vi "Slack-Dialog.vi"(0 "Cluster In":cluster{"Numeric":dbl}, 7 "AppName":string="Slack Demo") -> (4 "Cluster out":cluster{"Numeric":dbl}, 8 "Canceled?":bool)   [LabVIEW 2015]
uses:
  Controls/KBackground Gradient/KBackground Gradient.xctl
panel:
  in  "Gradient":dbl(xcontrol)
  in  "Tab":enum32{"Page 1", "Page 2"}(tab)
  out "Channel":string
  out "Workspace":string
  out "Users":i32(listbox) caption="channel"
  in  "Refresh Button":bool
  in  "Sign in Button":bool
  in  "Cancel":bool
  in  "OK":bool
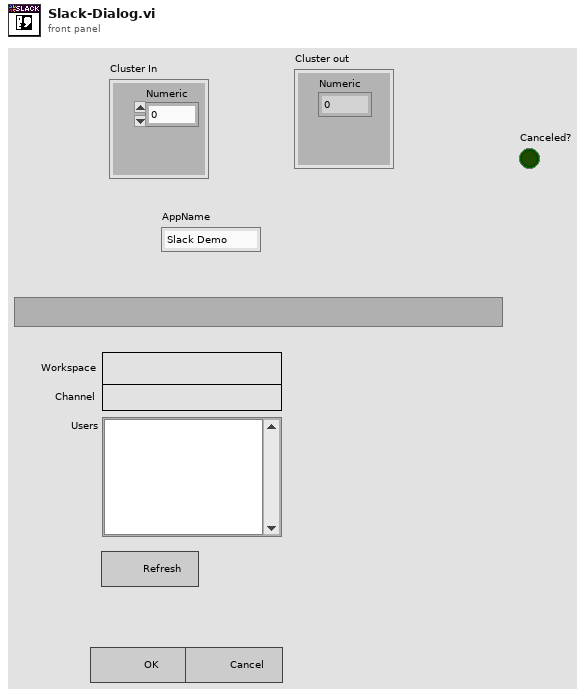
[diagram p1: front panel]
types:
  T1 = typedef "Slack-Configuration.ctl" = cluster{"app_id":string, "authed_user":cluster{"id":string}, "access_token":string, "bot_user_id":string, "team":cluster{"id":string, "name":string}, "bot channel":cluster{"id":string, "name":string}}
  T2 = typedef "Slack-User.ctl" = cluster{"id":string, "name":string}
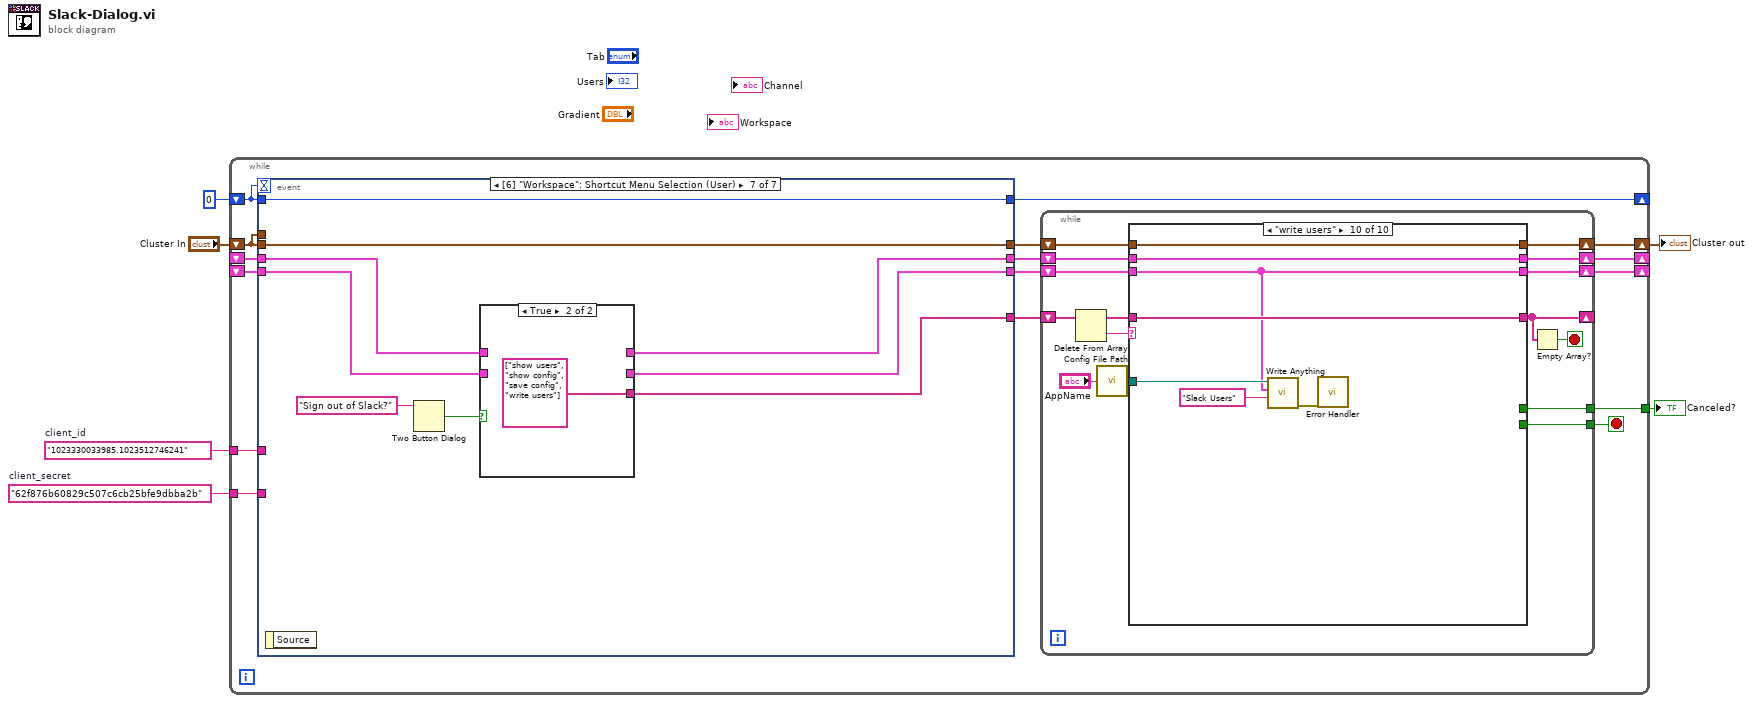
[diagram p0: block diagram]
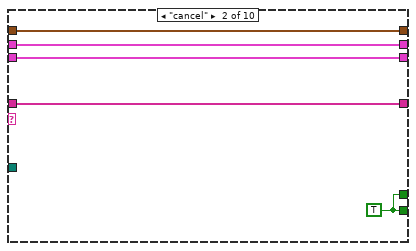
[diagram p3: hidden frame]
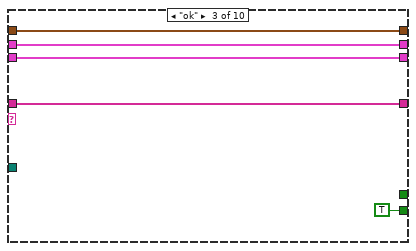
[diagram p4: hidden frame]
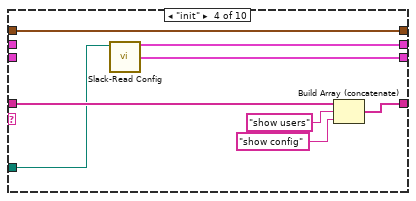
[diagram p5: hidden frame]
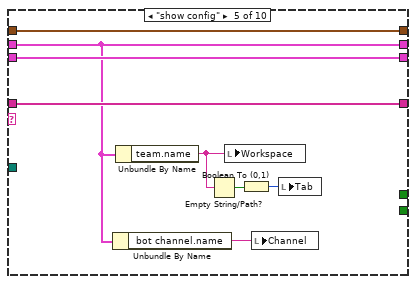
[diagram p6: hidden frame]
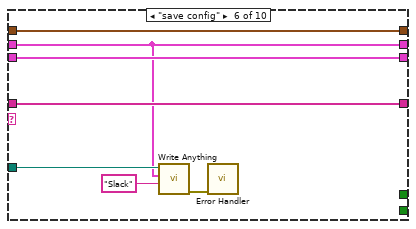
[diagram p7: hidden frame]
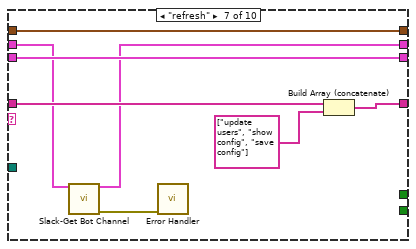
[diagram p8: hidden frame]
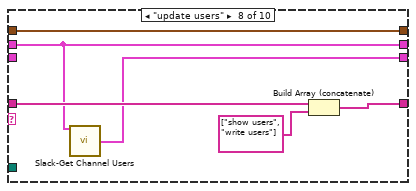
[diagram p9: hidden frame]
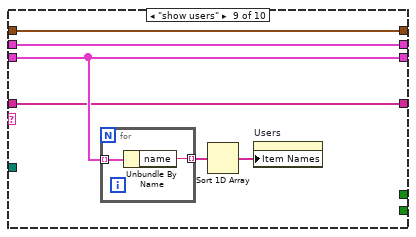
[diagram p10: hidden frame]
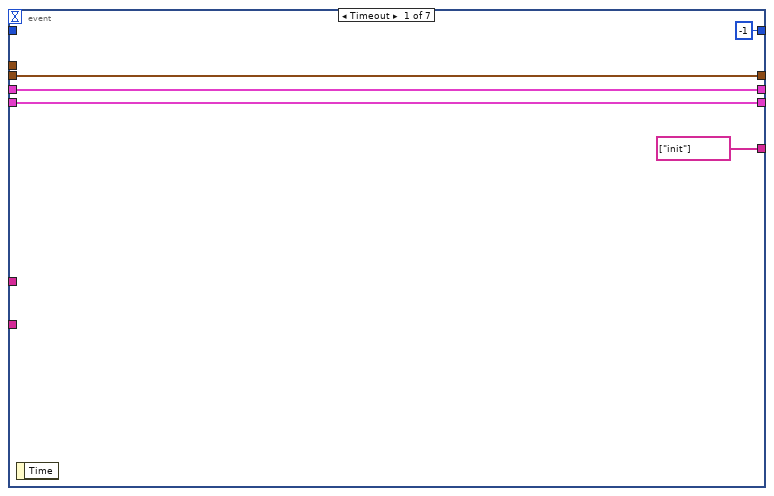
[diagram p11: hidden frame]
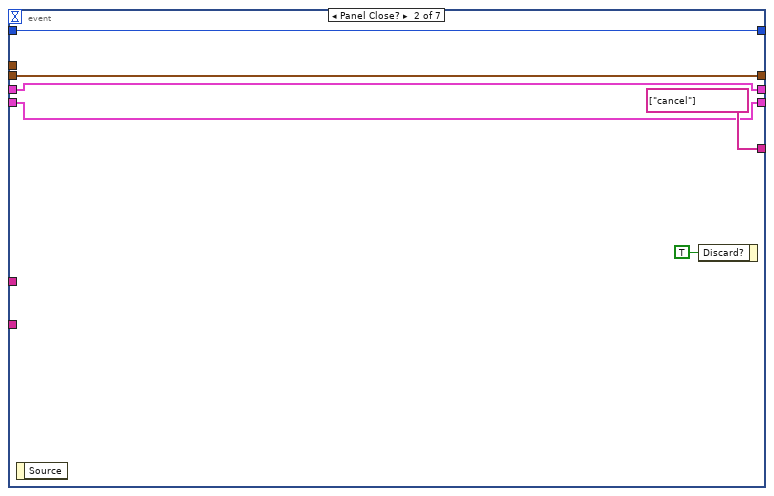
[diagram p12: hidden frame]
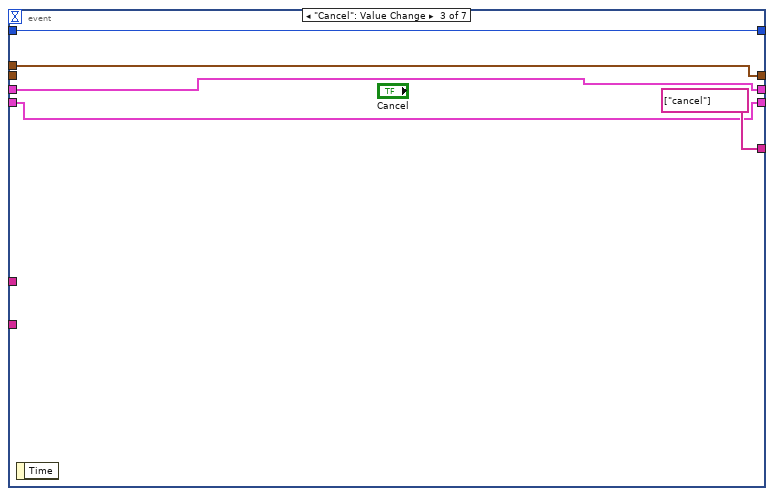
[diagram p13: hidden frame]
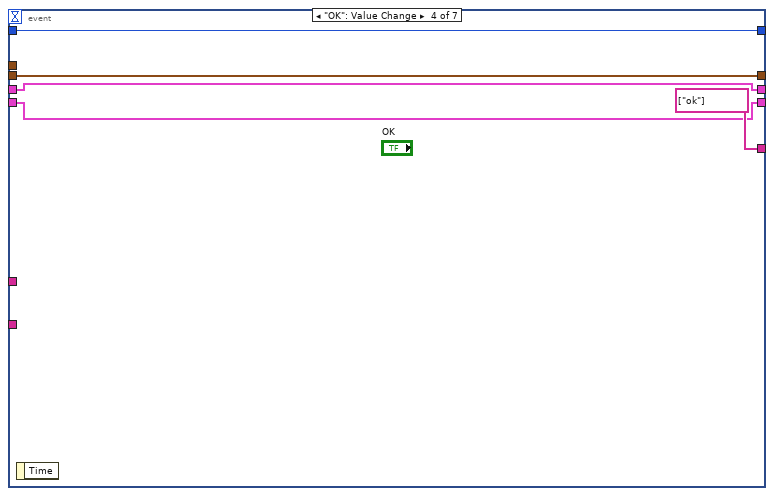
[diagram p14: hidden frame]
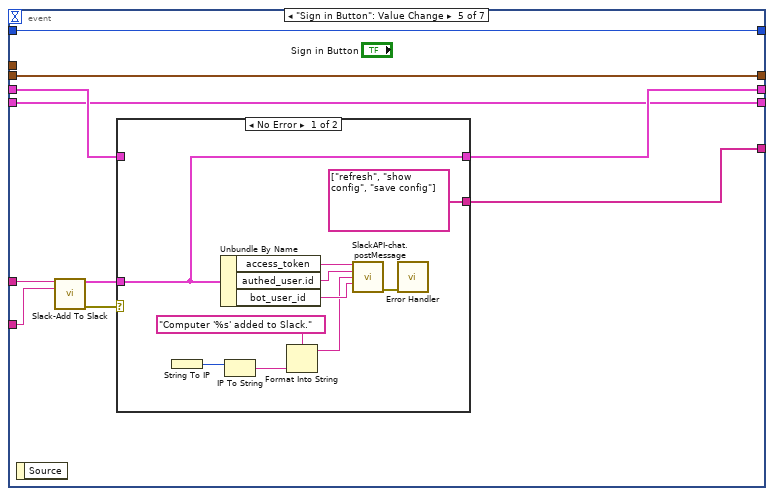
[diagram p15: hidden frame]
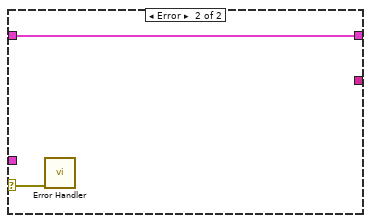
[diagram p16: hidden frame]
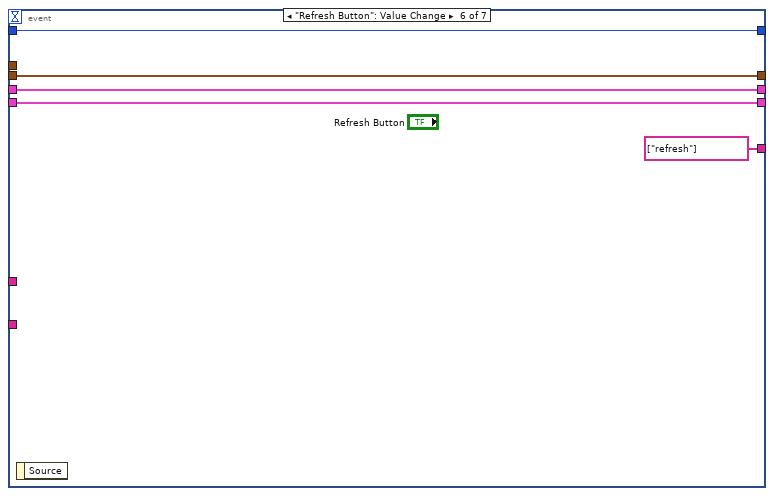
[diagram p17: hidden frame]
diagram:
  w1 = "62f876b60829c507c6cb25bfe9dbba2b"  # client_secret
  w2 = "1023330033985.1023512746241"  # client_id
  n1 = while {
    shift-right: [w22] -> _
    shift-left: 0 -> [w20]
    tunnel: [w15] -> w3
    shift-right: [w16] -> w4
    shift-left: "Cluster In" -> [w21]
    shift-right: [w14] -> _
    shift-left: _ -> [w12]
    shift-right: [w11] -> _
    shift-left: _ -> [w9]
    tunnel: w2 -> [w8]
    tunnel: w1 -> [w7]
    stop <- w17 stop-if-true
    n2 = event shown="[6] \"Workspace\": Shortcut Menu Selection (User)" {
      selector: _ -> [_ _ _ _ _ _ _]
      dyn-events: _ -> [_ _ _ _ _ _ _]
      timeout: w20 -> [_ _ _ _ _ _ _]
      tunnel: [-1 w114 w118 w123 w134 w151 w160] -> w22
      tunnel: w21 -> [w107 w113 _ w124 w133 w150 w159]
      tunnel: [w107 w113 w119 w124 w133 w150 w159] -> w19
      tunnel: w21 -> [_ _ w119 _ _ _ _]
      tunnel: w20 -> [_ w114 w118 w123 w134 w151 w160]
      tunnel: [string[] ["init"] string[] ["cancel"] string[] ["cancel"] string[] ["ok"] w125 string[] ["refresh"] w152] -> w18
      tunnel: [w105 w110 w116 w121 w129 w149 w155] -> w13
      tunnel: w12 -> [w105 w110 w116 w121 w128 w149 w156]
      tunnel: [w104 w109 w115 w120 w126 w148 w153] -> w10
      tunnel: w9 -> [w104 w109 w115 w120 w126 w148 w154]
      tunnel: w8 -> [_ _ _ _ w132 _ _]
      tunnel: w7 -> [_ _ _ _ w131 _ _]
      event Timeout {
        n3 = event-data() -> ()  [unwired: 1 in, 1 out]
      }
      event Panel Close? {
        n4 = event-data() -> ()  [unwired: 1 in, 1 out]
        n5 = event-data("Discard?"=TRUE) -> ()  [unwired: 1 in, 1 out]
      }
      event "Cancel": Value Change {
        n6 = event-data() -> ()  [unwired: 1 in, 1 out]
      }
      event "OK": Value Change {
        n7 = event-data() -> ()  [unwired: 1 in, 1 out]
      }
      event "Sign in Button": Value Change {
        n8 = event-data() -> ()  [unwired: 1 in, 1 out]
        n9 = call "Slack-Add To Slack.vi"("client_id"=w132, "client_secret"=w131) -> ("config"=w127:T1, "error out"=w130:errorcluster)  [unwired: 12 in]
        n10 = case shown="No Error" w130 {
          selector: w130 -> [_ w145]
          tunnel: [w140 w146] -> w129
          tunnel: w128 -> [_ w146]
          tunnel: w127 -> [w140 _]
          tunnel: [string[] ["refresh", "show config", "save config"] _] -> w125
          frame No Error {
            n11 = String To IP() -> (0:w143:u32)  [unwired: 1 in]
            n12 = Unbundle By Name(w140) -> ("access_token"=w139:string, "authed_user.id"=w138:string, "bot_user_id"=w137:string)
            n13 = IP To String(2:w143) -> (0:w141:string)  [unwired: 1 in]
            n14 = Format Into String(format string="Computer '%s' added to Slack.", w141) -> (resulting string=w136:string)  [unwired: 2 in, 1 out]
            n15 = call "SlackAPI-chat.postMessage.vi"("access_token"=w139, "user ID"=w138, "message"=w136, "username"=w137) -> ("error out"=w135:errorcluster)  [unwired: 11 in]
            n16 = call "Error Handler.vi"("error in (no error)"=w135) -> ()  [unwired: 13 in, 2 out]
          }
          frame Error {
            n17 = call "Error Handler.vi"("error in (no error)"=w145) -> ()  [unwired: 13 in, 2 out]
          }
        }
      }
      event "Refresh Button": Value Change {
        n18 = event-data() -> ()  [unwired: 1 in, 1 out]
      }
      event "Workspace": Shortcut Menu Selection (User) {
        n19 = event-data() -> ()  [unwired: 1 in, 1 out]
        n20 = Two Button Dialog(message="Sign out of Slack?" ("T button name (\"OK\")")) -> (T button?=w157:bool)  [unwired: 2 in]
        n21 = case shown="True" w157 {
          tunnel: w154 -> [w161 _]
          tunnel: w156 -> [w162 _]
          tunnel: [w162 _] -> w155
          tunnel: [w161 _] -> w153
          tunnel: [_ string[] ["show users", "show config", "save config", "write users"]] -> w152
          frame False {
          }
          frame True {
          }
        }
      }
    }
    n22 = while {
      shift-right: [w24] -> _
      shift-left: w18 -> [w37]
      shift-right: [w32] -> w16
      shift-left: w19 -> [w33]
      tunnel: [w31] -> w17
      tunnel: [w30] -> w15
      shift-right: [w29] -> w14
      shift-left: w13 -> [w28]
      shift-right: [w27] -> w11
      shift-left: w10 -> [w26]
      stop <- w34 stop-if-true
      n23 = Delete From Array(array=w37) -> (deleted portion=w35:string, array with subset deleted=w36:string[])  [unwired: 2 in]
      n24 = call "Config File Path.vi"("AppName"="AppName") -> ("Default config file name"=w23:path)
      n25 = case shown="\"write users\"" w35 {
        tunnel: w36 -> [w38 w42 w47 w59 w67 w74 w82 w88 w89 w103]
        tunnel: [w38 w42 w47 w56 w67 w74 w76 w86 w89 w103] -> w24
        tunnel: w33 -> [w41 w46 w51 w58 w66 w73 w81 w87 w94 w102]
        tunnel: [w41 w46 w51 w58 w66 w73 w81 w87 w94 w102] -> w32
        tunnel: [_ w45 TRUE _ _ _ _ _ _ _] -> w31
        tunnel: [_ w45 _ _ _ _ _ _ _ _] -> w30
        tunnel: [w40 w44 w49 w52 w61 w69 w77 w84 w91 w101] -> w29
        tunnel: w28 -> [w40 w44 w49 _ w61 w69 w78 w84 w91 w101]
        tunnel: [w39 w43 w48 w57 w62 w72 w80 w83 w90 w99] -> w27
        tunnel: w26 -> [w39 w43 w48 _ w62 w72 w80 _ w90 w99]
        tunnel: w23 -> [_ _ _ w54 _ w70 _ _ _ w100]
        frame "", Default {
        }
        frame "cancel" {
          w45 = TRUE
        }
        frame "ok" {
        }
        frame "init" {
          n26 = call "Slack-Read Config.vi"("AppName"=w54) -> ("config"=w52:T1, "Users"=w57:T2[])  [unwired: 12 in, 1 out]
          n27 = Build Array (concatenate)(w59, "show users", "show config") -> (w56:string[])
        }
        frame "show config" {
          n28 = Unbundle By Name(w61) -> ("bot channel.name"=w60:string)
          n29 = Unbundle By Name(w61) -> ("team.name"=w64:string)
          n30 = Empty String/Path?(string/path=w64) -> (empty?=w63:bool)
          n31 = local write "Workspace"(w64) -> ()
          n32 = Boolean To (0,1)(Boolean=w63) -> (0, 1=w65:i16)
          n33 = local write "Channel"(w60) -> ()
          n34 = local write "Tab"(w65) -> ()
        }
        frame "save config" {
          n35 = call "Write Anything.vi"("Section Name (Name of \"Anything\")"="Slack" ("Section Name (Name of \"Anything\")"), "Anything"=w69, "Path (dialog)"=w70) -> ("Error Out"=w68:errorcluster)  [unwired: 7 in, 1 out]
          n36 = call "Error Handler.vi"("error in (no error)"=w68) -> ()  [unwired: 13 in, 2 out]
        }
        frame "refresh" {
          n37 = call "Slack-Get Bot Channel.vi"("config in"=w78) -> ("config out"=w77:T1, "error out"=w79:errorcluster)  [unwired: 13 in]
          n38 = call "Error Handler.vi"("error in (no error)"=w79) -> ()  [unwired: 13 in, 2 out]
          n39 = Build Array (concatenate)(w82, string[] ["update users", "show config", "save config"]) -> (w76:string[])
        }
        frame "update users" {
          n40 = call "Slack-Get Channel Users.vi"("config in"=w84) -> ("users"=w83:T2[])  [unwired: 13 in, 1 out]
          n41 = Build Array (concatenate)(w88, string[] ["show users", "write users"]) -> (w86:string[])
        }
        frame "show users" {
          n42 = for {
            tunnel: w90 -> [w96] mode=indexing
            tunnel: [w95] -> w93 mode=indexing
            n43 = Unbundle By Name(w96) -> ("name"=w95:string)
          }
          n44 = Sort 1D Array(array=w93) -> (sorted array=w92:string[])
          n45 = property on="Users" class="LstBox (strict)"("Item Names"=w92) -> ()  [unwired: 2 in, 2 out]
        }
        frame "write users" {
          n46 = call "Write Anything.vi"("Section Name (Name of \"Anything\")"="Slack Users" ("Section Name (Name of \"Anything\")"), "Anything"=w99, "Path (dialog)"=w100) -> ("Error Out"=w97:errorcluster)  [unwired: 7 in, 1 out]
          n47 = call "Error Handler.vi"("error in (no error)"=w97) -> ()  [unwired: 13 in, 2 out]
        }
      }
      n48 = Empty Array?(array=w24) -> (empty?=w34:bool)
    }
  }
  "Cluster out" <- w4
  "Canceled?" <- w3
